vi "FeedbackDecode_RecordAV.vi"(3 "FullDataPath":path=path "D:/00000000-000000") -> ()   [LabVIEW 2020]
doc: "The Low-Level Grab VI configures the number of buffers to use for the acquisition and configures an event callback to handle every other acquired image. A grab is appropriate for high-speed applications in which you need to process only one image at a time."
uses:
  <vilib>/vision/Image Controls.llb/IMAQ Image.ctl
  <vilib>/userDefined/High Color/IMAQdx.ctl
  <vilib>/vision/Avi.llb/IMAQ AVI2 Refnum.ctl
  <vilib>/sound2/lvsound2.llb/Sound File Refnum.ctl
  <vilib>/sound2/lvsound2.llb/Sound Data Format.ctl
  <vilib>/vision/driver/IMAQdx.llb/IMAQdx Acquisition Mode.ctl
  <vilib>/vision/driver/IMAQdx.llb/IMAQdx Buffer Number Mode.ctl
  <vilib>/DAQmx/read.llb/DAQmx Read (Analog 2D DBL NChan NSamp).vi
  FeedbackDecode_Globals.vi
  <vilib>/sound2/lvsound2.llb/Sound File Write Open.vi
  <vilib>/DAQmx/miscellaneous.llb/DAQmx Fill In Error Info.vi
  <vilib>/sound2/lvsound2.llb/Sound File Write (DBL Single).vi
  <vilib>/vision/driver/NI_Vision_Acquisition_Software.lvlib
  <resource>/objmgr/imaqdx.rc
panel:
  out "AudTask":refnum<k21>
  out "FileTime":string
  out "AudBuffSize":i32=44100
  in  "AudParams":T1={"sample rate (S/s)"=44100.0, "number of channels"=1, "bits per sample"=16}
  out "AudReadSize":i32
  out "VidTask":T2
  out "WAVRef":T3
  out "AVIRef":T4
  out "FrmEvnt":refnum<event-registration>
  out "BufferImg":T5
  out "StopAud":bool
  out "StopVid":bool
  out "StitchResult":string
  out "WAVName":path
  out "AVIName":path
  out "DataFolderName":string="00000000-000000"
  out "FrameRate":dbl
  out "WAVChart":dbl[](graph)
  out "WAVLoopTime":u32(graph)=555
  out "SkippedFrames":i32
  out "FrameCount":i32
  out "AVILoopTime":u32(graph)=37
  out "AVIImage":T5(plugin-control)
  out "BufferNumber":u32
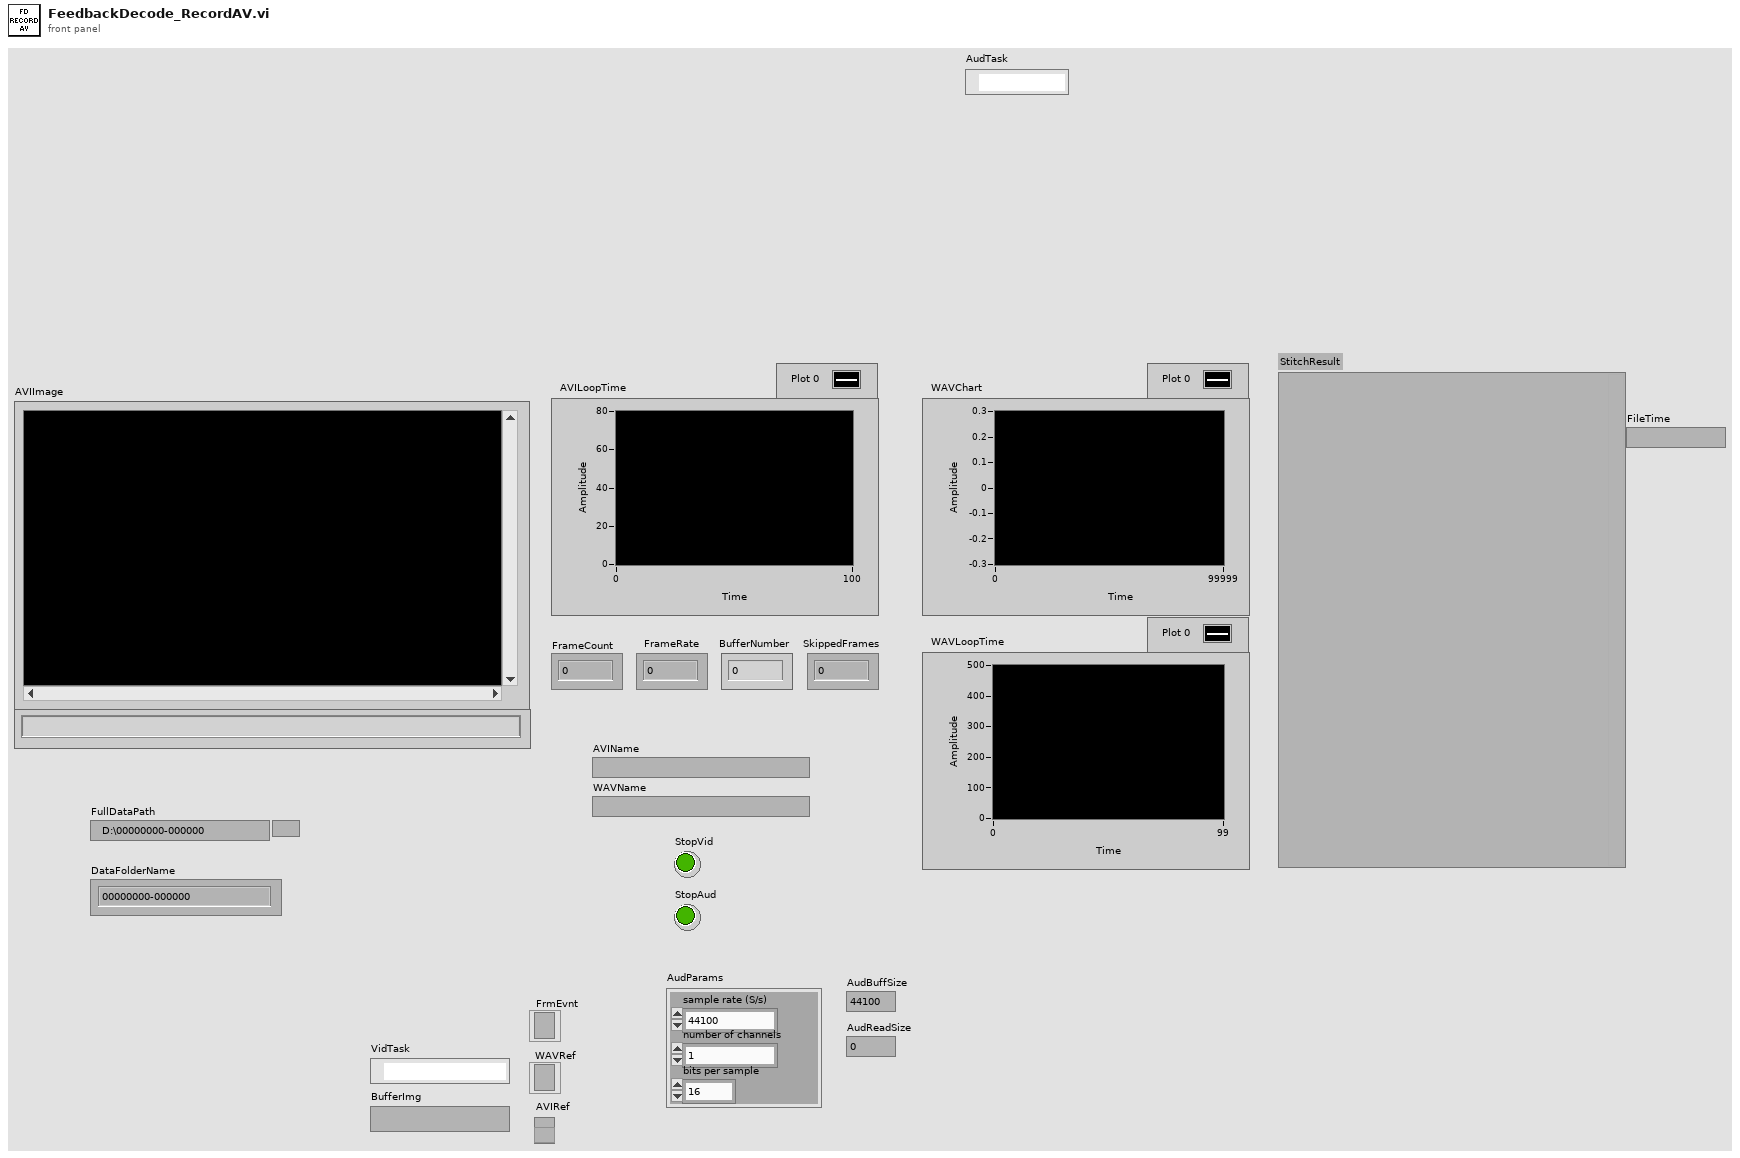
[diagram p1: front panel]
types:
  T1 = typedef "Sound Data Format.ctl" = cluster{"sample rate (S/s)":dbl, "number of channels":i32, "bits per sample":i32}
  T2 = typedef "IMAQdx.ctl" = refnum<k21>
  T3 = typedef "Sound File Refnum.ctl" = refnum<file>
  T4 = typedef "IMAQ AVI2 Refnum.ctl" = refnum<k20>
  T5 = typedef "IMAQ Image.ctl" = refnum<image>
  T6 = typedef "NI_Vision_Acquisition_Software.lvlib/IMAQdx Acquisition Mode.ctl" = enum32{"One Shot", "Continuous"}
  T7 = typedef "NI_Vision_Acquisition_Software.lvlib/IMAQdx Buffer Number Mode.ctl" = enum32{"Next", "Last", "Buffer Number", "Every", "Last New"}
  T8 = cluster{"Video Mode":u32, "Video Mode Name":string}[]
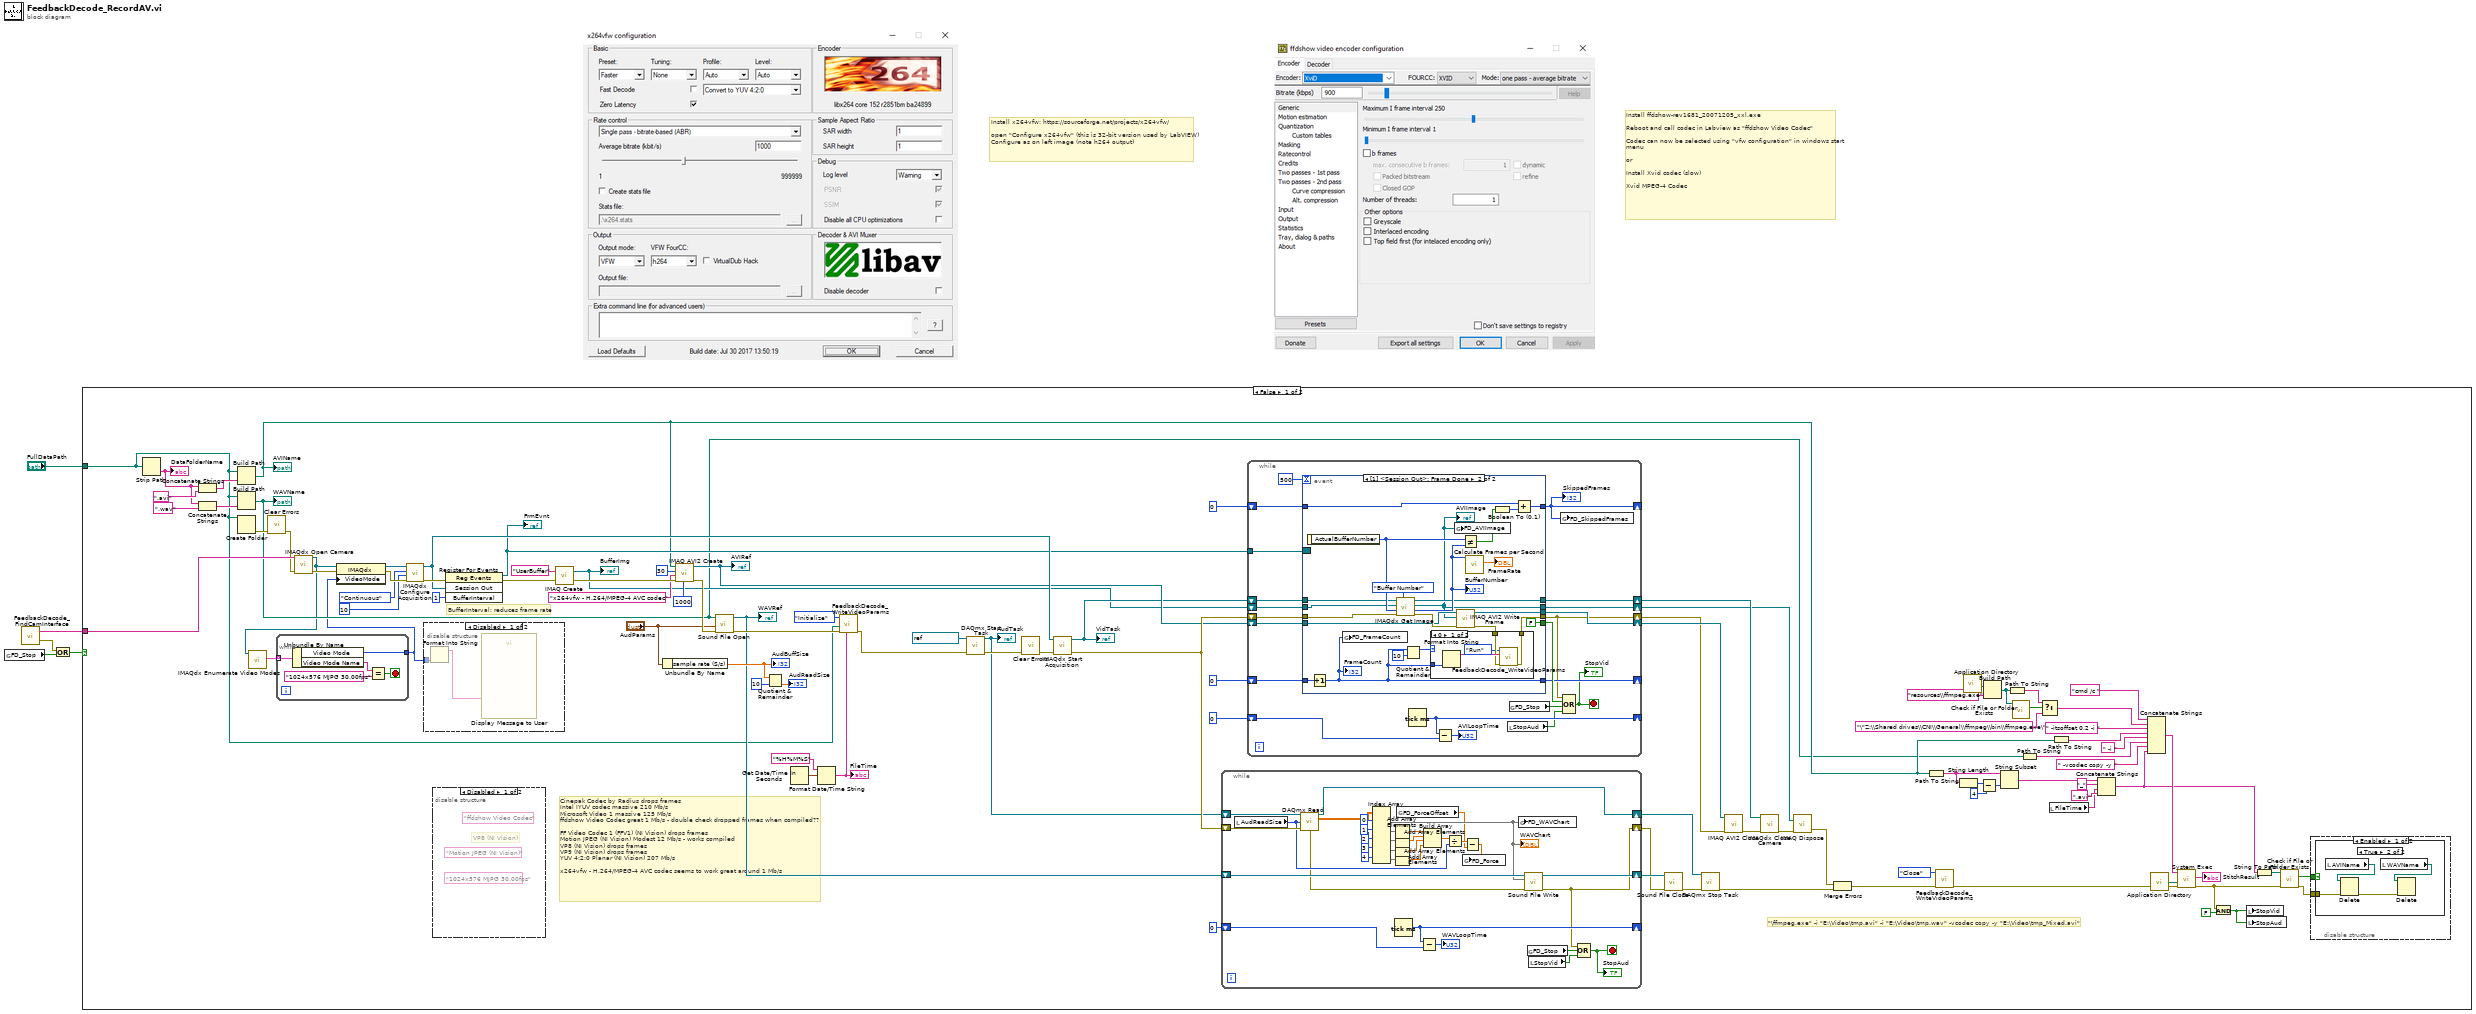
[diagram p0: block diagram]
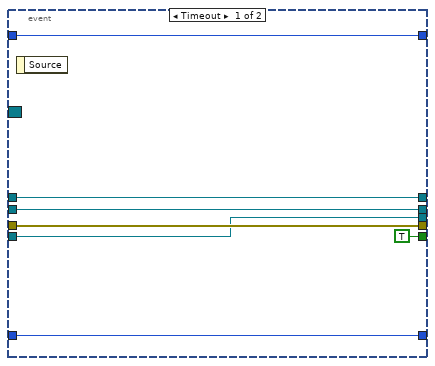
[diagram p6: hidden frame]
diagram:
  # "Install x264vfw: https://sourceforge.net/projects/x264vfw/ \n\nopen \"Configure x264vfw\" (this is 32-bit version used by LabVIEW)\nConfigure as on left image (note h264 output)"
  # "Install ffdshow-rev1681_20071205_xxl.exe\n\nReboot and call codec in Labview as \"ffdshow Video Codec\"\n\nCodec can now be selected using \"vfw configuration\" in windows start menu\n\nor\n\nInstall Xvid codec (slow)\n\nXvid MPEG-4 Codec"
  n1 = global read "FeedbackDecode_Globals.vi" "FD_Stop"() -> (w4:bool)
  n2 = call "FeedbackDecode_FindCamInterface.vi"() -> ("ErrorOut"=w2:errorcluster, "CamInterface"=w5:string)  [unwired: 2 in]
  n3 = Or(x=w2, y=w4) -> (x .or. y?=w3:bool)
  n4 = case shown="False" w3 {
    tunnel: w5 -> [w101 _]
    tunnel: "FullDataPath" -> [w20 _]
    frame False {
      # "Cinepak Codec by Radius drops frames\nIntel IYUV codec massive 210 Mb/s\nMicrosoft Video 1 massive 125 Mb/s\nffdshow Video Codec great 1 Mb/s - double check dropped frames when compiled??\n    \nFF Video Codec 1 (FFV1) (NI Vision) drops frames\nMotion JPEG (NI Vision) Modest 12 Mb/s - works compiled\nVP8 (NI Vision) drops frames\nVP9 (NI Vision) drops frames\nYUV 4:2:0 Planar (NI Vision) 207 Mb/s\n\nx264vfw - H.264/MPEG-4 AVC codec seems to work great around 1 Mb/s"
      # "\"\\ffmpeg.exe\" -i \"E:\\Video\\tmp.avi\" -i \"E:\\Video\\tmp.wav\" -vcodec copy -y \"E:\\Video\\tmp_Mixed.avi\""
      # "BufferInterval: reduces frame rate"
      n5 = Strip Path(path=w20) -> (name=w49:string)  [unwired: 1 out]
      "DataFolderName" <- w49
      n6 = Concatenate Strings(w49, ".avi" ("string")) -> (w53:string)
      n7 = Concatenate Strings(w49, ".wav" ("string")) -> (w54:string)
      n8 = Build Path(base path=w20, name or relative path=w53) -> (appended path=w19:path)
      "AVIName" <- w19
      n9 = Build Path(base path=w20, name or relative path=w54) -> (appended path=w18:path)
      "WAVName" <- w18
      n10 = Create Folder(path (use dialog)=w20) -> (error out=w50:errorcluster)  [unwired: 2 in, 2 out]
      n11 = call <vilib>:"Clear Errors.vi"("error in (no error)"=w50) -> ("error out"=w48:errorcluster)  [unwired: 5 in, 1 out]
      n12 = call <vilib>:"IMAQdx Open Camera.vi"("error in"=w48, "Session In"=w101) -> ("error out"=w102:errorcluster, "Session Out"=w8:T2)  [unwired: 1 in, 7 out]
      n13 = call <vilib>:"IMAQdx Enumerate Video Modes.vi"("Session In"=w8) -> ("Video Modes"=w7:T8)  [unwired: 7 in, 3 out]
      n14 = while {
        tunnel: w7 -> [w117] mode=indexing
        tunnel: [w113] -> w6
        stop <- w114 stop-if-true
        n15 = Unbundle By Name(w117) -> ("Video Mode"=w113:u32, "Video Mode Name"=w116:string)
        n16 = Equal?(x=w116, y="1024x576 MJPG 30.00fps") -> (x = y?=w114:bool)
      }
      n17 = property class="IMAQdx"(reference=w8, error in=w102, "VideoMode"=w6) -> (reference out=w104:T2, error out=w103:errorcluster)
      n18 = call <vilib>:"IMAQdx Configure Acquisition.vi"("error in"=w103, "Number of Buffers"=u32 10 ("InternalBufferNumber"), "Continuous?"=IMAQdx_Acquisition_Mode."Continuous", "Session In"=w104) -> ("error out"=w97:errorcluster, "Session Out"=w46:T2)  [unwired: 6 out]
      n19 = disable-structure shown="Disabled" {
        disable-tunnel: w6 -> [w112 _]
        frame Disabled {
          n20 = Format Into String(w112) -> (resulting string=w111:string)  [unwired: 3 in, 1 out]
          n21 = call "Display Message to User"("Message"=w111) -> ()  [unwired: 9 in, 2 out]
        }
        frame Enabled {
        }
      }
      n22 = disable-structure shown="Disabled" {
        frame Disabled {
          (unwired) "1024x576 MJPG 30.00fps" ("y")
          (unwired) "Motion JPEG (NI Vision)" ("Codec")
          (unwired) "ffdshow Video Codec" ("Codec")
          # "VP8 (NI Vision)"
        }
        frame Enabled {
        }
      }
      n23 = register-events(error in=w97, w46, u32 1 ("BufferInterval")) -> (reference out=w29:refnum<event-registration>, error out=w99:errorcluster)  [unwired: 1 in]
      "FrmEvnt" <- w29
      n24 = call "IMAQ Create"("Image Name"="UserBuffer", "error in (no error)"=w99) -> ("New Image"=w27:T5, "error out"=w100:errorcluster)  [unwired: 2 in, 1 out]
      "BufferImg" <- w27
      n25 = Unbundle By Name("AudParams") -> ("sample rate (S/s)"=w87:dbl)
      "AudBuffSize" <- w87
      n26 = call "IMAQ AVI2 Create"("Quality"=1000, "error in (no error)"=w100, "Codec"="x264vfw - H.264/MPEG-4 AVC codec", "Frames Per Second"=u32 30, "AVI Path"=w19) -> ("error out"=w90:errorcluster, "AVI Refnum"=w33:T4)  [unwired: 5 in]
      "AVIRef" <- w33
      n27 = call-poly <vilib>:"Sound File Open.vi"("error in (no error)"=w90, "sound format"="AudParams", "path"=w18) -> ("error out"=w91:errorcluster, "sound file refnum"=w31:T3)  [unwired: 7 in]
      "WAVRef" <- w31
      n28 = Quotient & Remainder(x=w87, y=10) -> (floor(x/y)=→"AudReadSize":dbl)  [unwired: 1 out]
      n29 = Get Date/Time In Seconds() -> (seconds since 1Jan1904=w40:timestamp)
      n30 = Format Date/Time String(time format string (%c)="%H%M%S", seconds (now)=w40) -> (date/time string=w21:string)  [unwired: 1 in]
      "FileTime" <- w21
      n31 = call "FeedbackDecode_WriteVideoParams.vi"("FileTime"=w21, "ErrorIn"=w91, "DataPath"=w20, "Mode"=enum16{"Initialize", "Run", "Close"}."Initialize") -> ("ErrorOut"=w16:errorcluster)  [unwired: 6 in, 1 out]
      n32 = call <vilib>:"DAQmx Start Task.vi"("task/channels in"=refnum<k21> "aud_force", "error in"=w16) -> ("task out"=w14:refnum<k21>, "error out"=w15:errorcluster)  [unwired: 12 in]
      "AudTask" <- w14
      n33 = call <vilib>:"Clear Errors.vi"("error in (no error)"=w15) -> ("error out"=w85:errorcluster)  [unwired: 5 in, 1 out]
      n34 = call <vilib>:"IMAQdx Start Acquisition.vi"("error in"=w85, "Session In"=w46) -> ("error out"=w60:errorcluster, "Session Out"=w28:T2)  [unwired: 8 out]
      "VidTask" <- w28
      n35 = while {
        shift-right: [w150] -> _
        shift-left: u32 0 ("millisecond timer value") -> [w149]
        shift-right: [w143] -> w30
        shift-left: w31 -> [w144]
        shift-right: [w126] -> w13
        shift-left: w14 -> [w131]
        shift-right: [w142] -> w23
        shift-left: w60 -> [w130]
        stop <- w147 stop-if-true
        n36 = local read "AudReadSize"() -> (w129:i32)
        n37 = call-poly <vilib>:"DAQmx Read.vi"("task/channels in"=w131, "number of samples per channel"=w129, "error in"=w130) -> ("task out"=w126:refnum<k21>, "data"=w132:dbl[][], "error out"=w128:errorcluster)  [unwired: 10 in]
        n38 = Index Array(array=w132, index (row) #1=0 ("index (row)"), index (row) #2=1 ("index (row)"), index (row) #3=2 ("index (row)"), index (row) #4=3 ("index (row)"), index (row) #5=4 ("index (row)")) -> (element #1=w127:dbl[], element #2=w133:dbl[], element #3=w134:dbl[], element #4=w135:dbl[], element #5=w136:dbl[])  [unwired: 5 in]
        "WAVChart" <- w127
        n39 = Add Array Elements(numeric array=w133) -> (sum=w138:dbl)
        n40 = Add Array Elements(numeric array=w134) -> (sum=w137:dbl)
        n41 = Add Array Elements(numeric array=w135) -> (sum=w139:dbl)
        n42 = Add Array Elements(numeric array=w136) -> (sum=w140:dbl)
        n43 = Tick Count (ms)() -> (millisecond timer value=w150:u32)
        n44 = global read "FeedbackDecode_Globals.vi" "FD_ForceOffset"() -> (w124:dbl)
        n45 = Subtract(x=w150, y=w149) -> (x-y=→"WAVLoopTime":u32)
        n46 = Build Array(w138, w137, w139, w140) -> (w141:dbl[])
        n47 = Divide(x=w141, y=w129) -> (x/y=w125:dbl[])
        n48 = Subtract(x=w125, y=w124) -> (x-y=w123:dbl[])
        n49 = global write "FeedbackDecode_Globals.vi" "FD_Force"(w123) -> ()
        n50 = global write "FeedbackDecode_Globals.vi" "FD_WAVChart"(w127) -> ()
        n51 = call-poly <vilib>:"Sound File Write.vi"("error in (no error)"=w128, "data"=w127, "sound file refnum"=w144) -> ("error out"=w142:errorcluster, "sound file refnum out"=w143:T3)  [unwired: 7 in]
        n52 = global read "FeedbackDecode_Globals.vi" "FD_Stop"() -> (w145:bool)
        n53 = local read "StopVid"() -> (w146:bool)
        n54 = Compound Arithmetic op=OR(w142, w145, w146) -> (w147:bool)
        "StopAud" <- w147
      }
      n55 = while {
        shift-right: [w168] -> _
        shift-left: u32 0 ("millisecond timer value") -> [w167]
        shift-right: [w164] -> _
        shift-left: 0 -> [w165]
        shift-right: [w159] -> _
        shift-left: 0 -> [w163]
        shift-right: [w157] -> w32
        shift-left: w33 -> [w158]
        tunnel: w29 -> [w156]
        shift-right: [w154] -> w26
        shift-left: w28 -> [w155]
        shift-right: [w152] -> w25
        shift-left: w27 -> [w153]
        shift-right: [w151] -> w24
        shift-left: w60 -> [w171]
        stop <- w162 stop-if-true
        n56 = event shown="[1] <Session Out>: Frame Done" {
          selector: w156 -> [_ _]
          dyn-events: _ -> [_ _]
          timeout: 500 -> [_ _]
          tunnel: w171 -> [w176 w201]
          tunnel: [w176 w186] -> w151
          tunnel: [TRUE FALSE] -> w169
          tunnel: w165 -> [w178 w195]
          tunnel: [w178 w185] -> w164
          tunnel: w163 -> [w177 w192]
          tunnel: [w177 w191] -> w159
          tunnel: w158 -> [w174 w184]
          tunnel: [w174 w183] -> w157
          tunnel: w155 -> [w173 w182]
          tunnel: [w173 w181] -> w154
          tunnel: w153 -> [w172 w180]
          tunnel: [w172 w179] -> w152
          event Timeout {
            n57 = event-data() -> ()  [unwired: 2 out]
          }
          event event #0x0 {
            n58 = event-data() -> ("ActualBufferNumber"=w199:u32)  [unwired: 1 out]
            n59 = Increment(x=w195) -> (x+1=w185:i32)
            "FrameCount" <- w185
            n60 = global write "FeedbackDecode_Globals.vi" "FD_FrameCount"(w185) -> ()
            n61 = call <vilib>:"IMAQdx Get Image.vi"("Buffer Number Mode (Next)"=IMAQdx_Buffer_Number_Mode."Buffer Number" ("Buffer Number Mode"), "error in"=w201, "Buffer Number In"=w199, "Image In"=w180, "Session In"=w182) -> ("error out"=w198:errorcluster, "Buffer Number Out"=w196:u32, "Image Out"=w179:T5, "Session Out"=w181:T2)  [unwired: 3 in]
            "BufferNumber" <- w196
            "AVIImage" <- w179
            n62 = Quotient & Remainder(x=w185, y=10) -> (x-y*floor(x/y)=w188:i32)  [unwired: 1 out]
            n63 = global write "FeedbackDecode_Globals.vi" "FD_AVIImage"(w179) -> ()
            n64 = call "IMAQ AVI2 Write Frame"("error in (no error)"=w198, "Image"=w179, "AVI Refnum"=w184) -> ("error out"=w187:errorcluster, "AVI Refnum (duplicate)"=w183:T4)  [unwired: 6 in, 1 out]
            n65 = case shown="0" w188 {
              tunnel: w185 -> [w206 _]
              tunnel: w187 -> [w204 w207]
              tunnel: [w203 w207] -> w186
              frame 0 {
                n66 = Format Into String(w206) -> (resulting string=w205:string)  [unwired: 3 in, 1 out]
                n67 = call "FeedbackDecode_WriteVideoParams.vi"("ErrorIn"=w204, "Frame"=w205, "Mode"=enum16{"Initialize", "Run", "Close"}."Run") -> ("ErrorOut"=w203:errorcluster)  [unwired: 7 in, 1 out]
              }
              frame 1, Default {
              }
            }
            n68 = Not Equal?(x=w199, y=w196) -> (x != y?=w194:bool)
            n69 = call <vilib>:"Calculate Frames per Second.vi"("Buffer Number"=w196) -> ("Processed Frames/s"=→"FrameRate":dbl)  [unwired: 8 in, 2 out]
            n70 = Boolean To (0,1)(Boolean=w194) -> (0, 1=w193:i16)
            n71 = Add(x=w192, y=w193) -> (x+y=w191:i32)
          }
        }
        "SkippedFrames" <- w159
        n72 = Tick Count (ms)() -> (millisecond timer value=w168:u32)
        n73 = Subtract(x=w168, y=w167) -> (x-y=→"AVILoopTime":u32)
        n74 = local read "StopAud"() -> (w161:bool)
        n75 = global read "FeedbackDecode_Globals.vi" "FD_Stop"() -> (w160:bool)
        n76 = global write "FeedbackDecode_Globals.vi" "FD_SkippedFrames"(w159) -> ()
        n77 = Compound Arithmetic op=OR(w151, w169, w160, w161) -> (w162:bool)
        "StopVid" <- w162
      }
      n78 = call <vilib>:"Sound File Close.vi"("error in (no error)"=w23, "sound file refnum"=w30) -> ("error out"=w35:errorcluster)  [unwired: 9 in]
      n79 = call <vilib>:"DAQmx Stop Task.vi"("task/channels in"=w13, "error in"=w35) -> ("error out"=w34:errorcluster)  [unwired: 12 in, 1 out]
      n80 = call "IMAQ AVI2 Close"("error in (no error)"=w24, "AVI Refnum"=w32) -> ("error out"=w37:errorcluster)  [unwired: 9 in]
      n81 = call <vilib>:"IMAQdx Close Camera.vi"("error in"=w37, "Session In"=w26) -> ("error out"=w67:errorcluster)  [unwired: 9 out]
      n82 = call "IMAQ Dispose"("Image"=w25, "error in (no error)"=w67) -> ("error out"=w36:errorcluster)  [unwired: 4 in]
      n83 = Merge Errors(w36, w34) -> (w10:errorcluster)
      n84 = Path To String(path=w19) -> (string=w72:string)
      n85 = call "FeedbackDecode_WriteVideoParams.vi"("ErrorIn"=w10, "Mode"=enum16{"Initialize", "Run", "Close"}."Close") -> ("ErrorOut"=w9:errorcluster)  [unwired: 8 in, 1 out]
      n86 = String Length(string=w72) -> (length=w70:i32)
      n87 = call <vilib>:"Application Directory.vi"() -> ("Application Directory"=w77:path)
      n88 = Subtract(x=w70, y=4) -> (x-y=w71:i32)
      n89 = Build Path(base path=w77, name or relative path="resources\\ffmpeg.exe") -> (appended path=w45:path)
      n90 = String Subset(string=w72, length (rest)=w71) -> (substring=w73:string)  [unwired: 1 in]
      n91 = Path To String(path=w45) -> (string=w43:string)
      n92 = call <vilib>:"Check if File or Folder Exists.vi"("path"=w45) -> ("file or folder exists?"=w44:bool)  [unwired: 8 in, 2 out]
      n93 = Path To String(path=w18) -> (string=w76:string)
      n94 = Select(t=w43, s=w44, f="\"Z:\\Shared drives\\CNI\\General\\ffmpeg\\bin\\ffmpeg.exe\"" ("name or relative path")) -> (s? t:f=w41:string)
      n95 = local read "FileTime"() -> (w22:string)
      n96 = Path To String(path=w19) -> (string=w74:string)
      n97 = Concatenate Strings(w73, "_" ("string"), w22, ".avi" ("string")) -> (w59:string)
      n98 = Concatenate Strings("cmd /c ", w41, " -itsoffset 0.2 -i ", w74, " -i " ("string"), w76, " -vcodec copy -y " ("string"), w59) -> (w63:string)
      n99 = call <vilib>:"Application Directory.vi"() -> ("Application Directory"=w75:path)
      n100 = call <vilib>:"System Exec.vi"("error in (no error)"=w9, "working directory"=w75, "command line"=w63) -> ("error out"=w57:errorcluster, "standard error"=→"StitchResult":string)  [unwired: 5 in, 2 out]
      n101 = And(x=w57, y=FALSE) -> (x .and. y?=w68:bool)
      n102 = local write "StopVid"(w68) -> ()
      n103 = local write "StopAud"(w68) -> ()
      n104 = String To Path(string=w59) -> (path=w58:path)
      n105 = call <vilib>:"Check if File or Folder Exists.vi"("error in (no error)"=w57, "path"=w58) -> ("error out"=w56:errorcluster, "file or folder exists?"=w55:bool)  [unwired: 7 in, 1 out]
      n106 = disable-structure shown="Enabled" {
        disable-tunnel: w56 -> [w106 _]
        disable-tunnel: w55 -> [w105 _]
        frame Enabled {
          n107 = case shown="True" w105 {
            tunnel: w106 -> [_ w107]
            frame False {
            }
            frame True {
              n108 = local read "AVIName"() -> (w110:path)
              n109 = Delete(path (use dialog)=w110, error in=w107) -> (error out=w108:errorcluster)  [unwired: 3 in, 2 out]
              n110 = local read "WAVName"() -> (w109:path)
              n111 = Delete(path (use dialog)=w109, error in=w108) -> ()  [unwired: 3 in, 3 out]
            }
          }
        }
        frame Disabled {
        }
      }
    }
    frame True {
    }
  }
